vi "Refresh Frames to Sysdef Frames.vi"(8 "error in":errorcluster, 10 "Refresh Frames":T3[](array[typedef])) -> (0 "error out":errorcluster, 2 "Sysdef Frames":T1[](array[typedef]))   [LabVIEW 2020, in "Communication Bus Template System Explorer.lvlib" / "Implementation.lvlib"]
uses:
  Types/Frame.ctl
  Types/Signal.ctl
  Implementation.lvlib
  Types/Refresh Frame.ctl
  Types/Refresh Signal.ctl
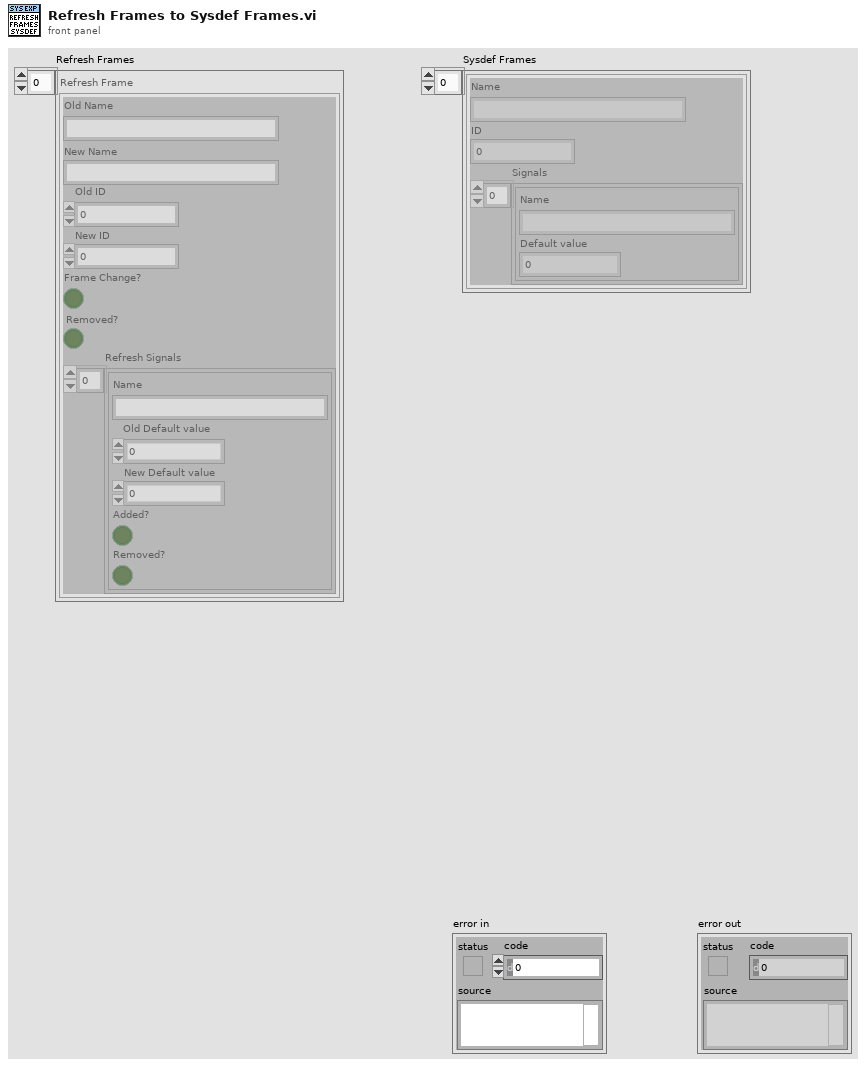
[diagram p1: front panel]
types:
  T1 = typedef "Communication Bus Template System Explorer.lvlib/Implementation.lvlib/Frame.ctl" = cluster{"Name":string, "ID":u32, "Signals":T2[]}
  T2 = typedef "Communication Bus Template System Explorer.lvlib/Implementation.lvlib/Signal.ctl" = cluster{"Name":string, "Default value":dbl}
  T3 = typedef "Communication Bus Template System Explorer.lvlib/Implementation.lvlib/Refresh Frame.ctl" = cluster{"Old Name":string, "New Name":string, "Old ID":u32, "New ID":u32, "Frame Change?":bool, "Removed?":bool, "Refresh Signals":T4[]}
  T4 = typedef "Communication Bus Template System Explorer.lvlib/Implementation.lvlib/Refresh Signal.ctl" = cluster{"Name":string, "Old Default value":dbl, "New Default value":dbl, "Added?":bool, "Removed?":bool}
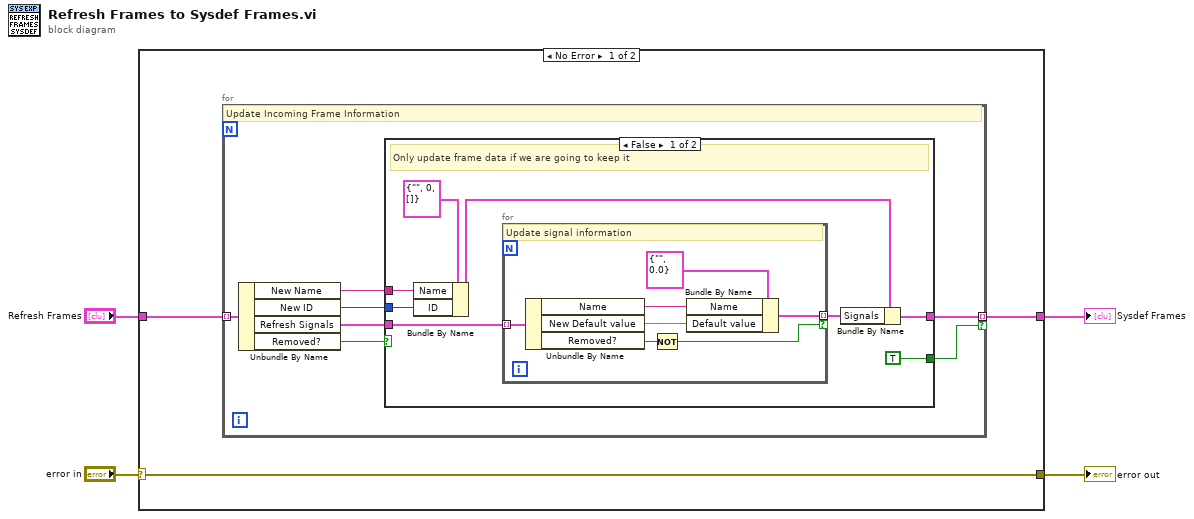
[diagram p0: block diagram]
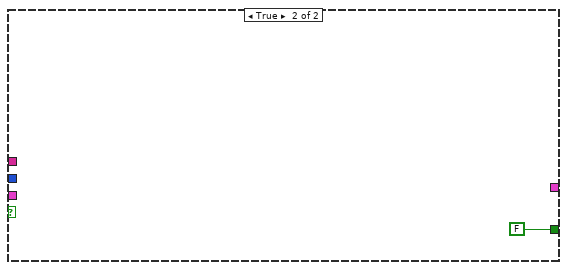
[diagram p2: hidden frame]
diagram:
  n1 = case shown="No Error" "error in" {
    selector: "error in" -> [w7 w31]
    tunnel: [w5 _] -> w1
    tunnel: [w7 w31] -> w3
    tunnel: "Refresh Frames" -> [w6 _]
    frame No Error {
      n2 = for {
        tunnel: w6 -> [w14] mode=indexing
        tunnel: [w10] -> w5 mode=indexing if=w8
        # "Update Incoming Frame Information"
        n3 = Unbundle By Name(w14) -> ("New Name"=w13:string, "New ID"=w12:u32, "Refresh Signals"=w11:T4[], "Removed?"=w9:bool)
        n4 = case shown="False" w9 {
          tunnel: w13 -> [w21 _]
          tunnel: w12 -> [w20 _]
          tunnel: w11 -> [w19 _]
          tunnel: [w16 _] -> w10
          tunnel: [TRUE FALSE] -> w8
          frame False {
            # "Only update frame data if we are going to keep it"
            n5 = Bundle By Name(cluster=T1 {"Name"="", "ID"=0, "Signals"=[]} ("Frame"), "Name"=w21, "ID"=w20) -> (w18:T1)
            n6 = for {
              tunnel: w19 -> [w29] mode=indexing
              tunnel: [w27] -> w17 mode=indexing if=w23
              # "Update signal information"
              n7 = Unbundle By Name(w29) -> ("Name"=w26:string, "New Default value"=w25:dbl, "Removed?"=w24:bool)
              n8 = Not(x=w24) -> (.not. x?=w23:bool)
              n9 = Bundle By Name(cluster=T2 {"Name"="", "Default value"=0.0} ("Signal"), "Name"=w26, "Default value"=w25) -> (w27:T2)
            }
            n10 = Bundle By Name(cluster=w18, "Signals"=w17) -> (w16:T1)
          }
          frame True {
          }
        }
      }
    }
    frame Error {
    }
  }
  "error out" <- w3
  "Sysdef Frames" <- w1
